vi "TestVI.vi"(8 "y":dbl=6.0, 11 "x":dbl=20.0) -> (3 "x+y+1":dbl(slide) scale=0.0..100.0)   [LabVIEW 2023, in "Class2.lvclass"]
doc: "Output = x+y+1"
uses:
  Class2.lvclass
  Class2.lvclass/Class2.ctl
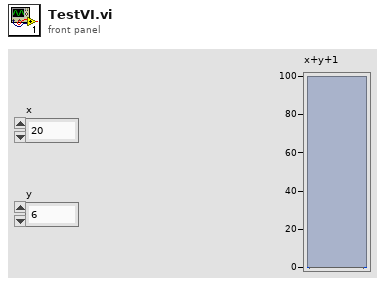
[diagram p1: front panel]
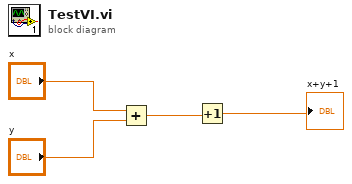
[diagram p0: block diagram]
diagram:
  n1 = Add(x="x", y="y") -> (x+y=w4:dbl)
  n2 = Increment(x=w4) -> (x+1=→"x+y+1":dbl)
